vi "Get Table Name.vi"(8 "error in (no error)":errorcluster caption="错误输入（无错误）", 11 "DataTable输入":refnum<class "DataTable.lvclass">) -> (0 "error out":errorcluster caption="错误输出", 2 "Table Name":string, 3 "DataTable输出":refnum<class "DataTable.lvclass">)   [LabVIEW 2012, in "Data Grid VIEW.lvlib" / "DataTable.lvclass"]
uses:
  DataTable.lvclass
  DataTable.lvclass/DataTable.ctl
  System.Data
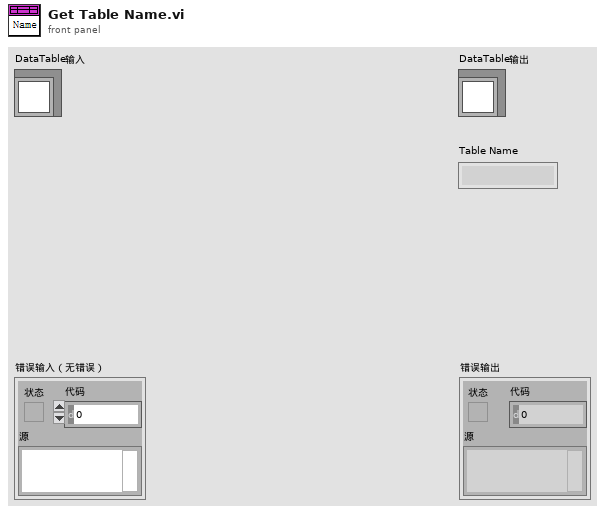
[diagram p1: front panel]
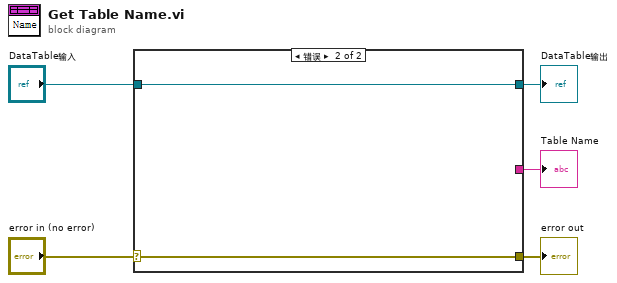
[diagram p0: block diagram]
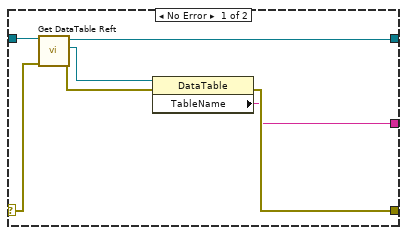
[diagram p2: hidden frame]
diagram:
  n1 = case shown="错误" "error in (no error)" {
    selector: "error in (no error)" -> [w11 w13]
    tunnel: [w8 w13] -> w4
    tunnel: [w6 w14] -> w3
    tunnel: "DataTable输入" -> [w12 w14]
    tunnel: [w7 _] -> w1
    frame No Error {
      n2 = call "Get DataTable Reft.vi"("error in (no error)"=w11, "DataTable输入"=w12) -> ("error out"=w9:errorcluster, "DataTable"=w10:refnum<k24>, "DataTable输出"=w6:refnum<class "DataTable.lvclass">)  [unwired: 7 in]
      n3 = property class="DataTable"(reference=w10, error in=w9) -> (error out=w8:errorcluster, "TableName"=w7:string)  [unwired: 1 out]
    }
    frame Error {
    }
  }
  "error out" <- w4
  "DataTable输出" <- w3
  "Table Name" <- w1
